vi "Start.vi"(8 "error in (no error)":errorcluster, 10 "Message in":refnum<class "StartMessage.lvclass">, 11 "TomoConversion in":refnum<class "TomoConversion.lvclass">) -> (0 "error out":errorcluster, 3 "TomoConversion out":refnum<class "TomoConversion.lvclass">)   [LabVIEW 2012, in "TomoConversion.lvclass"]
doc: "This member function is called when the statemachine in the run.vi receives an 'start' command. It relays the message to all observers of the component.\n\nOverride this member function in your derived class if you need additional start functionality (but don't forget to call the parent method)."
uses:
  TomoConversion.lvclass
  <vilib>/Distrio/Distrio/Murmex/StartMessage/StartMessage.lvclass
  <vilib>/Distrio/Distrio/Murmex/Murmex/Murmex.lvclass
  <vilib>/Distrio/Distrio/Murmex/ProceedMessage/ProceedMessage.lvclass
panel:
  # "This member function is called when the statemachine in the run.vi receives an 'start' command. It relays the message to all observers of the component.\n\nOverride this member function in your derived class if you need additional start functionality (but don't forget to call the parent method)."
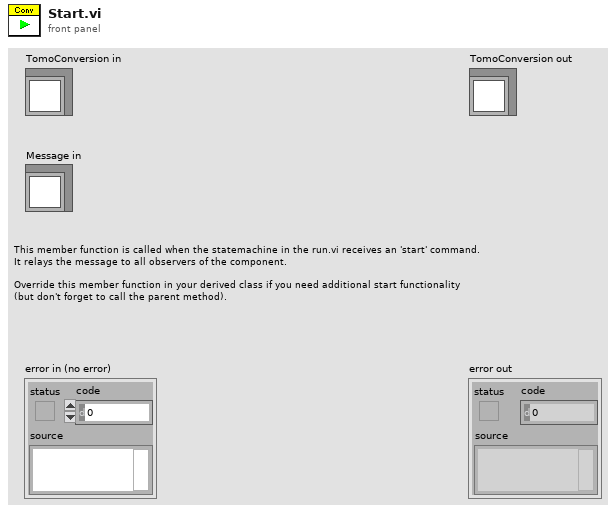
[diagram p1: front panel]
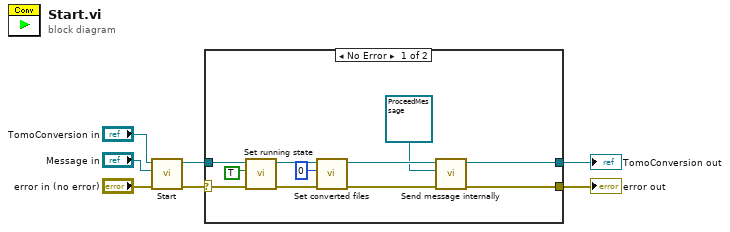
[diagram p0: block diagram]
diagram:
  n1 = call-parent "Start.vi"("error in (no error)"="error in (no error)", "Message in"="Message in", "Murmex in"="TomoConversion in") -> ("error out"=w4:errorcluster, "Murmex out"=w3:refnum<class "TomoConversion.lvclass">)  [unwired: 7 in]
  n2 = case shown="No Error" w4 {
    selector: w4 -> [w18 w19]
    tunnel: w3 -> [w16 w20]
    tunnel: [w11 w19] -> w2
    tunnel: [w9 w20] -> w1
    frame No Error {
      n3 = call-dynamic "Set running state.vi"("error in (no error)"=w18, "is running?"=TRUE, "TomoConversion in"=w16) -> ("error out"=w15:errorcluster, "TomoConversion out"=w13:refnum<class "TomoConversion.lvclass">)  [unwired: 7 in]
      n4 = call-dynamic "Set converted files.vi"("error in (no error)"=w15, "converted cxd files"=0, "TomoConversion in"=w13) -> ("error out"=w14:errorcluster, "TomoConversion out"=w10:refnum<class "TomoConversion.lvclass">)  [unwired: 7 in]
      n5 = call <vilib>:"Send message internally.vi"("error in (no error)"=w14, "Message"=refnum<class "ProceedMessage.lvclass"> refnum ("Distrio Murmex 1.2:ProceedMessage"), "Murmex in"=w10) -> ("error out"=w11:errorcluster, "Murmex out"=w9:refnum<class "TomoConversion.lvclass">)  [unwired: 7 in]
    }
    frame Error {
    }
  }
  "error out" <- w2
  "TomoConversion out" <- w1
